vi "test_remove_key_string.vi"(8 "error in (no error)":errorcluster) -> (0 "error out":errorcluster)   [LabVIEW 2020]
uses:
  9b058582-e2fa-4656-a80f-7a9f04272724.vi
  9b058582-e2fa-4656-a80f-7a9f04272724.vi/5c360ba9-55da-4dc8-b351-3905cb0f7927.vi
  9b058582-e2fa-4656-a80f-7a9f04272724.vi/97c372d5-b07b-4406-bdf7-223d7ecb307b.vi
  toml/delete_subtable_item.vi
  toml/toml.lvclass
  <vilib>/addons/_JKI Toolkits/Caraya/classes/Assert/Assert.lvclass
  <vilib>/addons/_JKI Toolkits/Caraya/classes/Test/Test.lvclass
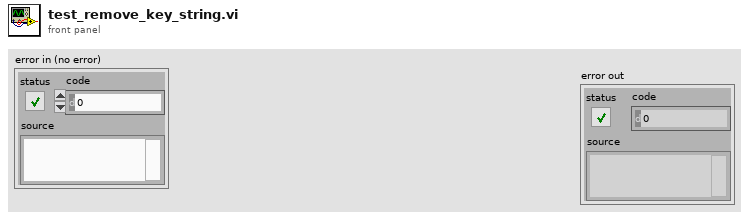
[diagram p1: front panel]
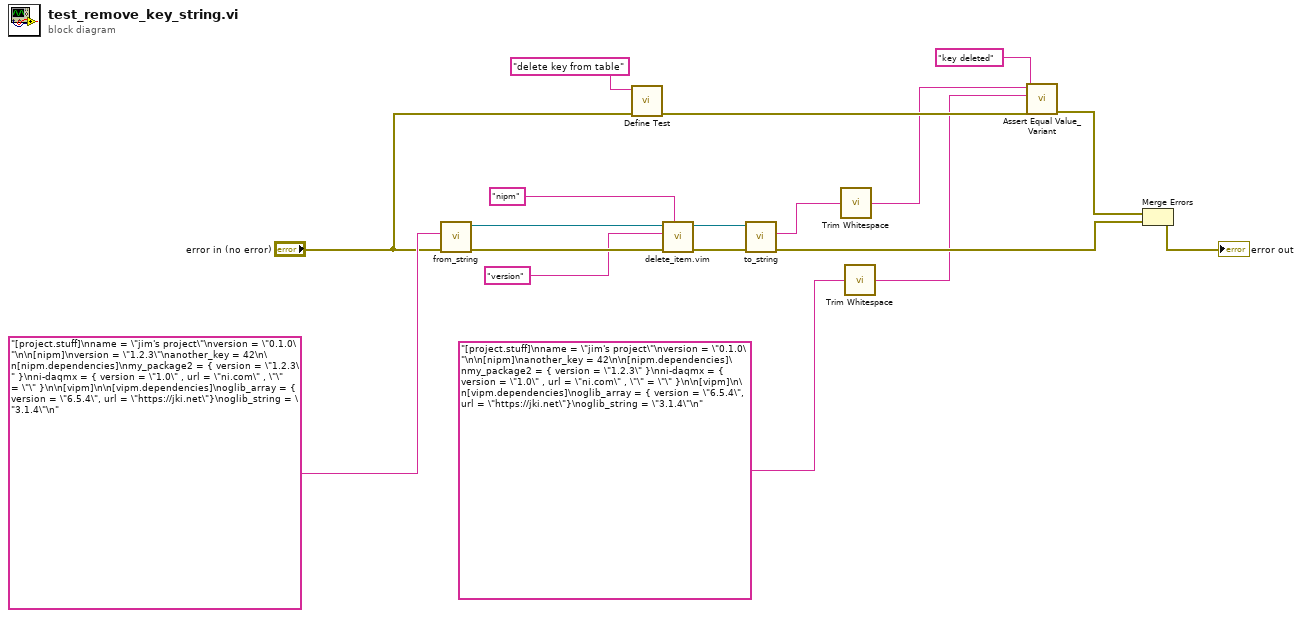
[diagram p0: block diagram]
diagram:
  n1 = call "from_string.vi"("error in (no error)"="error in (no error)", "toml"="[project.stuff]\nname = \"jim's project\"\nversion = \"0.1.0\"\n\n[nipm]\nversion = \"1.2.3\"\nanother_key = 42\n\n[nipm.dependencies]\nmy_package2 = { version = \"1.2.3\" }\nni-daqmx = { version = \"1.0\" , url = \"ni.com\" , \"\" = \"\" }\n\n[vipm]\n\n[vipm.dependencies]\noglib_array = { version = \"6.5.4\", url = \"https://jki.net\"}\noglib_string = \"3.1.4\"\n" ("toml_string in")) -> ("error out"=w15:errorcluster, "toml out"=w14:refnum<class "toml.lvclass">)  [unwired: 8 in]
  n2 = call <vilib>:"Define Test.vi"("error in (no error)"="error in (no error)", "Label (VI Title)"="delete key from table") -> ("error out"=w8:errorcluster)  [unwired: 9 in]
  n3 = call "delete_item.vim"("table (subtables)"="nipm" ("table_name"), "error in (no error)"=w15, "key (subkeys)"="version" ("table_name"), "toml in"=w14) -> ("error out"=w17:errorcluster, "toml out"=w16:refnum<class "toml.lvclass">)  [unwired: 5 in, 1 out]
  n4 = call "to_string.vi"("error in (no error)"=w17, "toml in"=w16) -> ("error out"=w11:errorcluster, "toml_string"=w6:string)  [unwired: 8 in]
  n5 = call <vilib>:"Trim Whitespace.vi"("string"=w6) -> ("trimmed string"=w5:string)  [unwired: 1 in]
  n6 = call <vilib>:"Trim Whitespace.vi"("string"="[project.stuff]\nname = \"jim's project\"\nversion = \"0.1.0\"\n\n[nipm]\nanother_key = 42\n\n[nipm.dependencies]\nmy_package2 = { version = \"1.2.3\" }\nni-daqmx = { version = \"1.0\" , url = \"ni.com\" , \"\" = \"\" }\n\n[vipm]\n\n[vipm.dependencies]\noglib_array = { version = \"6.5.4\", url = \"https://jki.net\"}\noglib_string = \"3.1.4\"\n" ("toml_string in")) -> ("trimmed string"=w3:string)  [unwired: 1 in]
  n7 = call <vilib>:"Assert Equal Value_Variant.vi"("Label"="key deleted", "error in (no error)"=w8, "Y"=w3, "X"=w5) -> ("error out"=w12:errorcluster)  [unwired: 7 in]
  n8 = Merge Errors(w12, w11) -> (→"error out":errorcluster)
